vi "VDCInputErrors.vi"(1 "Array":u16[](array[numeric])=[0, 0, 0, 0, 0, 0, 0, 0, 0, 0, 0, 0, 0, 0, 0, 0, 0, 0, 0, 0, 0, 0, 0, 0, 0, 0, 0, 0, 0, 0, 0, 0, 0, 0, 0, 0, 0, 0, 0, 0, 0, 0, 0, 0, 0, 0, 0, 0, 0, 0, 0, 0, 0, 0, 0, 0, 0, 0, 0, 0, 0, 0, 0, 0, 0, 0, 0, 0, 0, 0, 0, 0, 0, 0, 0, 0, 0, 0, 0, 0, 0, 0, 0, 0, 0, 0, 0, 0, 0, 0, 0, 0, 0, 0, 0, 0, 0, 0, 0, 0, 0, 0, 0, 0, 0, 0, 0, 0, 0, 0, 0, 0, 0, 0, 0, 0, 0, 0, 0, 0, 0, 0, 0, 0, 0, 0, 0, 0, 0, 0, 0, 0, 0, 0, 0, 0, 0, 0, 0, 0, 0, 0, 0, 0, 0, 0, 0, 0, 0, 0, 0, 0, 0, 0, 0, 0, 0, 0, 0, 0, 0, 0, 0, 0, 0, 0, 0, 0, 0, 0, 0, 0, 0, 0, 0, 0, 0, 0, 0, 0, 0]) -> (0 "output cluster":T1)   [LabVIEW 2017]
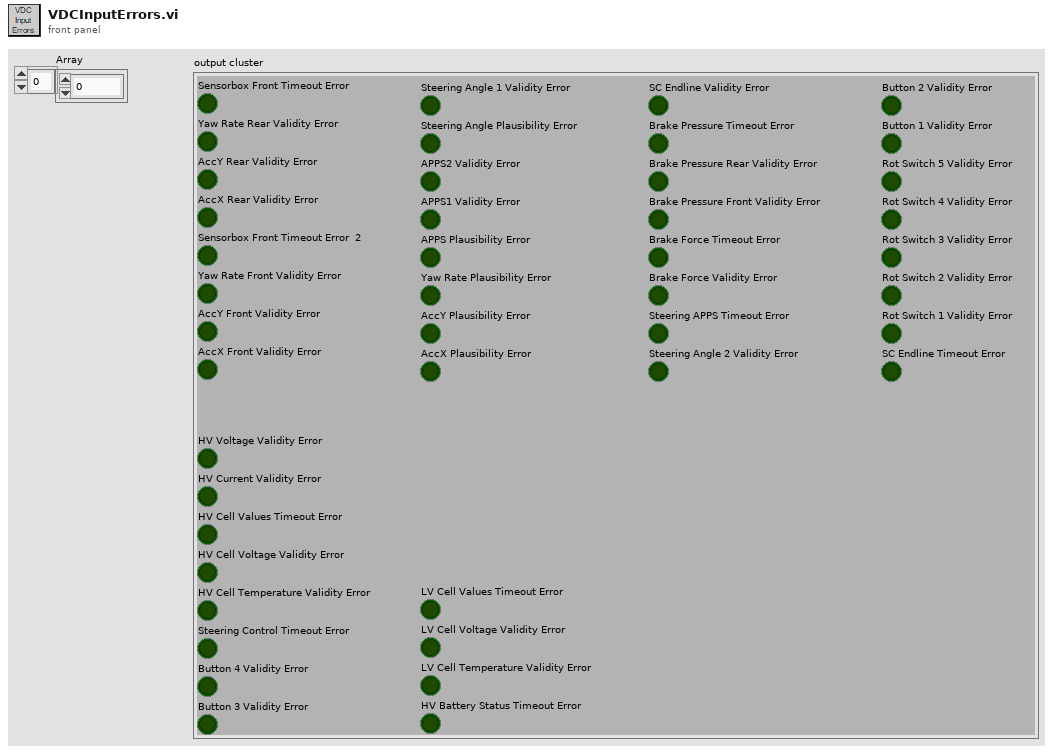
[diagram p1: front panel]
types:
  T1 = cluster{"Sensorbox Front Timeout Error ":bool, "Yaw Rate Rear Validity Error ":bool, "AccY Rear Validity Error":bool, "AccX Rear Validity Error ":bool, "Sensorbox Front Timeout Error  2":bool, "Yaw Rate Front Validity Error":bool, "AccY Front Validity Error":bool, "AccX Front Validity Error":bool, "Steering Angle 1 Validity Error":bool, "Steering Angle Plausibility Error":bool, "APPS2 Validity Error":bool, "APPS1 Validity Error":bool, "APPS Plausibility Error ":bool, "Yaw Rate Plausibility Error ":bool, "AccY Plausibility Error ":bool, "AccX Plausibility Error ":bool, "SC Endline Validity Error":bool, "Brake Pressure Timeout Error ":bool, "Brake Pressure Rear Validity Error":bool, "Brake Pressure Front Validity Error":bool, "Brake Force Timeout Error ":bool, "Brake Force Validity Error ":bool, "Steering APPS Timeout Error":bool, "Steering Angle 2 Validity Error":bool, "Button 2 Validity Error":bool, "Button 1 Validity Error":bool, "Rot Switch 5 Validity Error":bool, "Rot Switch 4 Validity Error":bool, "Rot Switch 3 Validity Error":bool, "Rot Switch 2 Validity Error":bool, "Rot Switch 1 Validity Error":bool, "SC Endline Timeout Error":bool, "HV Voltage Validity Error":bool, "HV Current Validity Error":bool, "HV Cell Values Timeout Error":bool, "HV Cell Voltage Validity Error":bool, "HV Cell Temperature Validity Error":bool, "Steering Control Timeout Error":bool, "Button 4 Validity Error":bool, "Button 3 Validity Error":bool, "LV Cell Values Timeout Error":bool, "LV Cell Voltage Validity Error":bool, "LV Cell Temperature Validity Error":bool, "HV Battery Status Timeout Error":bool}
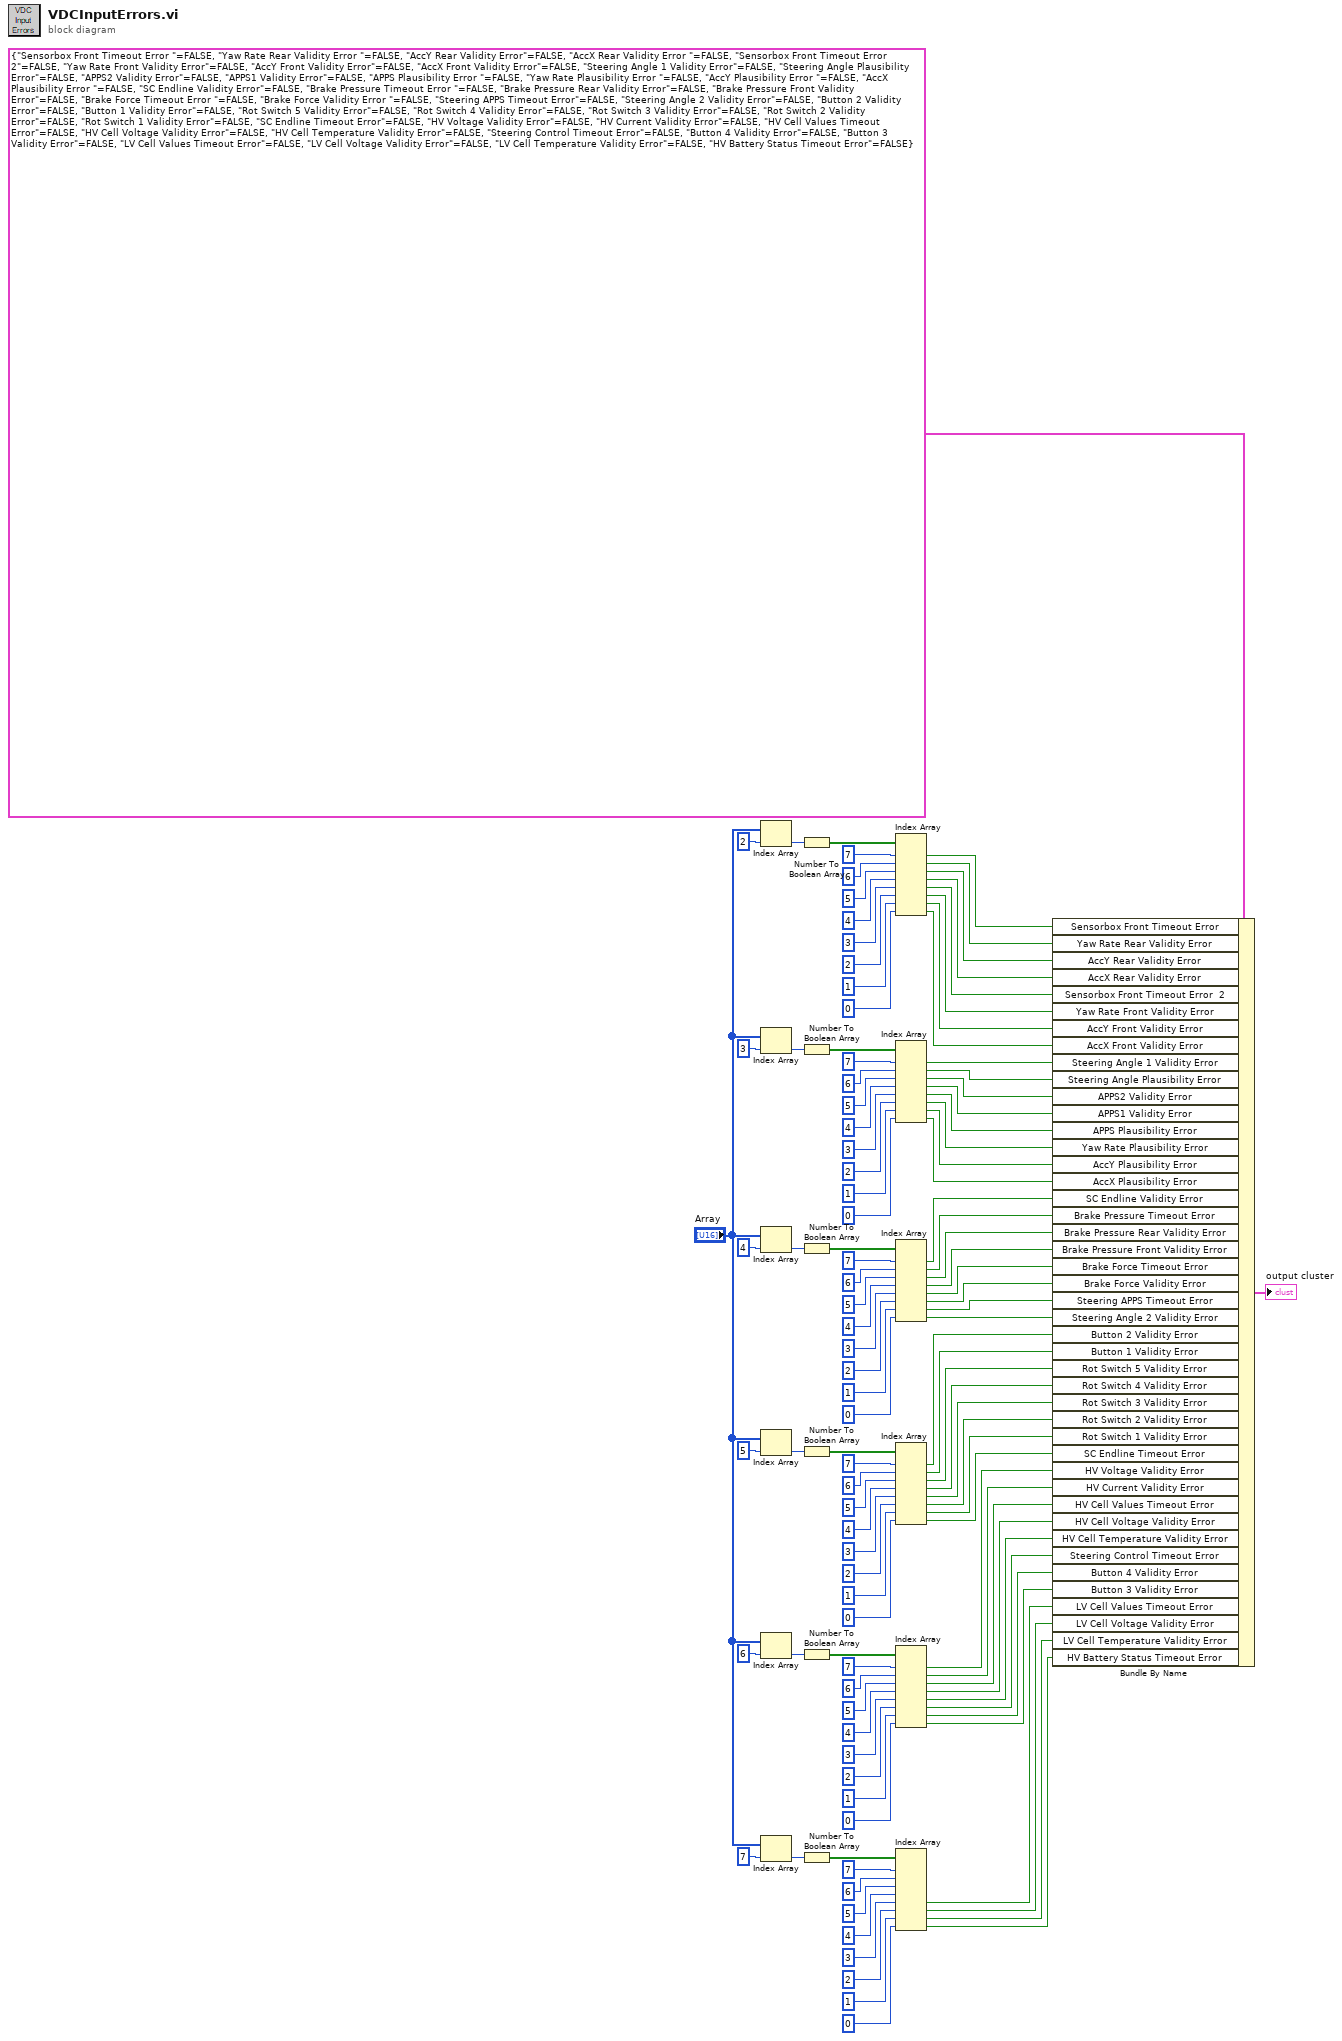
[diagram p0: block diagram]
diagram:
  n1 = Index Array(array="Array", index=2) -> (element=w81:u16)
  n2 = Index Array(array="Array", index=3) -> (element=w102:u16)
  n3 = Index Array(array="Array", index=4) -> (element=w103:u16)
  n4 = Index Array(array="Array", index=5) -> (element=w80:u16)
  n5 = Index Array(array="Array", index=6) -> (element=w61:u16)
  n6 = Index Array(array="Array", index=7) -> (element=w57:u16)
  n7 = Number To Boolean Array(number=w81) -> (Boolean array=w90:bool[])
  n8 = Number To Boolean Array(number=w102) -> (Boolean array=w93:bool[])
  n9 = Number To Boolean Array(number=w103) -> (Boolean array=w112:bool[])
  n10 = Number To Boolean Array(number=w80) -> (Boolean array=w71:bool[])
  n11 = Number To Boolean Array(number=w61) -> (Boolean array=w70:bool[])
  n12 = Number To Boolean Array(number=w57) -> (Boolean array=w48:bool[])
  n13 = Index Array(array=w90, index #1=7 ("index"), index #2=6 ("index"), index #3=5 ("index"), index #4=4 ("index"), index #5=3 ("index"), index #6=2 ("index"), index #7=1 ("index"), index #8=0 ("index")) -> (element #1=w45:bool, element #2=w44:bool, element #3=w43:bool, element #4=w42:bool, element #5=w41:bool, element #6=w40:bool, element #7=w39:bool, element #8=w38:bool)
  n14 = Index Array(array=w93, index #1=7 ("index"), index #2=6 ("index"), index #3=5 ("index"), index #4=4 ("index"), index #5=3 ("index"), index #6=2 ("index"), index #7=1 ("index"), index #8=0 ("index")) -> (element #1=w37:bool, element #2=w36:bool, element #3=w35:bool, element #4=w34:bool, element #5=w33:bool, element #6=w32:bool, element #7=w31:bool, element #8=w30:bool)
  n15 = Index Array(array=w112, index #1=7 ("index"), index #2=6 ("index"), index #3=5 ("index"), index #4=4 ("index"), index #5=3 ("index"), index #6=2 ("index"), index #7=1 ("index"), index #8=0 ("index")) -> (element #1=w29:bool, element #2=w28:bool, element #3=w27:bool, element #4=w26:bool, element #5=w25:bool, element #6=w24:bool, element #7=w23:bool, element #8=w22:bool)
  n16 = Index Array(array=w71, index #1=7 ("index"), index #2=6 ("index"), index #3=5 ("index"), index #4=4 ("index"), index #5=3 ("index"), index #6=2 ("index"), index #7=1 ("index"), index #8=0 ("index")) -> (element #1=w21:bool, element #2=w20:bool, element #3=w19:bool, element #4=w18:bool, element #5=w17:bool, element #6=w16:bool, element #7=w15:bool, element #8=w14:bool)
  n17 = Index Array(array=w70, index #1=7 ("index"), index #2=6 ("index"), index #3=5 ("index"), index #4=4 ("index"), index #5=3 ("index"), index #6=2 ("index"), index #7=1 ("index"), index #8=0 ("index")) -> (element #1=w13:bool, element #2=w12:bool, element #3=w11:bool, element #4=w10:bool, element #5=w9:bool, element #6=w8:bool, element #7=w7:bool, element #8=w6:bool)
  n18 = Index Array(array=w48, index #1=7 ("index"), index #2=6 ("index"), index #3=5 ("index"), index #4=4 ("index"), index #5=3 ("index"), index #6=2 ("index"), index #7=1 ("index"), index #8=0 ("index")) -> (element #5=w5:bool, element #6=w4:bool, element #7=w3:bool, element #8=w2:bool)  [unwired: 4 out]
  n19 = Bundle By Name(cluster=T1 {"Sensorbox Front Timeout Error "=FALSE, "Yaw Rate Rear Validity Error "=FALSE, "AccY Rear Validity Error"=FALSE, "AccX Rear Validity Error "=FALSE, "Sensorbox Front Timeout Error  2"=FALSE, "Yaw Rate Front Validity Error"=FALSE, "AccY Front Validity Error"=FALSE, "AccX Front Validity Error"=FALSE, "Steering Angle 1 Validity Error"=FALSE, "Steering Angle Plausibility Error"=FALSE, "APPS2 Validity Error"=FALSE, "APPS1 Validity Error"=FALSE, "APPS Plausibility Error "=FALSE, "Yaw Rate Plausibility Error "=FALSE, "AccY Plausibility Error "=FALSE, "AccX Plausibility Error "=FALSE, "SC Endline Validity Error"=FALSE, "Brake Pressure Timeout Error "=FALSE, "Brake Pressure Rear Validity Error"=FALSE, "Brake Pressure Front Validity Error"=FALSE, "Brake Force Timeout Error "=FALSE, "Brake Force Validity Error "=FALSE, "Steering APPS Timeout Error"=FALSE, "Steering Angle 2 Validity Error"=FALSE, "Button 2 Validity Error"=FALSE, "Button 1 Validity Error"=FALSE, "Rot Switch 5 Validity Error"=FALSE, "Rot Switch 4 Validity Error"=FALSE, "Rot Switch 3 Validity Error"=FALSE, "Rot Switch 2 Validity Error"=FALSE, "Rot Switch 1 Validity Error"=FALSE, "SC Endline Timeout Error"=FALSE, "HV Voltage Validity Error"=FALSE, "HV Current Validity Error"=FALSE, "HV Cell Values Timeout Error"=FALSE, "HV Cell Voltage Validity Error"=FALSE, "HV Cell Temperature Validity Error"=FALSE, "Steering Control Timeout Error"=FALSE, "Button 4 Validity Error"=FALSE, "Button 3 Validity Error"=FALSE, "LV Cell Values Timeout Error"=FALSE, "LV Cell Voltage Validity Error"=FALSE, "LV Cell Temperature Validity Error"=FALSE, "HV Battery Status Timeout Error"=FALSE}, "Sensorbox Front Timeout Error"=w45, "Yaw Rate Rear Validity Error"=w44, "AccY Rear Validity Error"=w43, "AccX Rear Validity Error"=w42, "Sensorbox Front Timeout Error  2"=w41, "Yaw Rate Front Validity Error"=w40, "AccY Front Validity Error"=w39, "AccX Front Validity Error"=w38, "Steering Angle 1 Validity Error"=w37, "Steering Angle Plausibility Error"=w36, "APPS2 Validity Error"=w35, "APPS1 Validity Error"=w34, "APPS Plausibility Error"=w33, "Yaw Rate Plausibility Error"=w32, "AccY Plausibility Error"=w31, "AccX Plausibility Error"=w30, "SC Endline Validity Error"=w29, "Brake Pressure Timeout Error"=w28, "Brake Pressure Rear Validity Error"=w27, "Brake Pressure Front Validity Error"=w26, "Brake Force Timeout Error"=w25, "Brake Force Validity Error"=w24, "Steering APPS Timeout Error"=w23, "Steering Angle 2 Validity Error"=w22, "Button 2 Validity Error"=w21, "Button 1 Validity Error"=w20, "Rot Switch 5 Validity Error"=w19, "Rot Switch 4 Validity Error"=w18, "Rot Switch 3 Validity Error"=w17, "Rot Switch 2 Validity Error"=w16, "Rot Switch 1 Validity Error"=w15, "SC Endline Timeout Error"=w14, "HV Voltage Validity Error"=w13, "HV Current Validity Error"=w12, "HV Cell Values Timeout Error"=w11, "HV Cell Voltage Validity Error"=w10, "HV Cell Temperature Validity Error"=w9, "Steering Control Timeout Error"=w8, "Button 4 Validity Error"=w7, "Button 3 Validity Error"=w6, "LV Cell Values Timeout Error"=w5, "LV Cell Voltage Validity Error"=w4, "LV Cell Temperature Validity Error"=w3, "HV Battery Status Timeout Error"=w2) -> (→"output cluster":T1)
